vi "IMAQdx Enumerate Video Modes.vi"(8 "error in":errorcluster, 11 "Session In":T1) -> (0 "error out":errorcluster, 1 "Current Mode":u32, 2 "Video Modes":T2(array[cluster]), 3 "Session Out":T1)   [LabVIEW 2020, in "NI_Vision_Acquisition_Software.lvlib"]
doc: "Returns a list of video modes supported by the camera."
uses:
  NI_Vision_Acquisition_Software.lvlib
  IMAQdx.ctl
  niimaqdx.dll
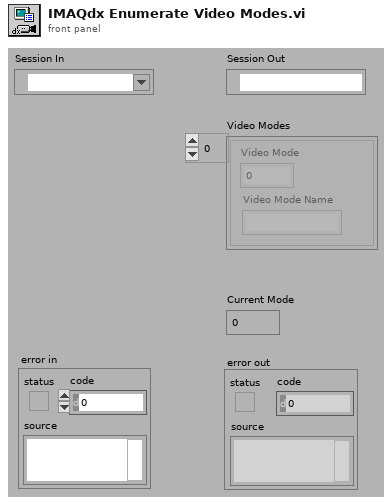
[diagram p1: front panel]
types:
  T1 = typedef "IMAQdx.ctl" = refnum<k21>
  T2 = cluster{"Video Mode":u32, "Video Mode Name":string}[]
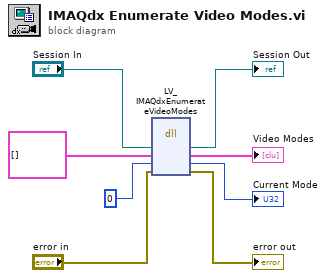
[diagram p0: block diagram]
diagram:
  n1 = dll-call lib="niimaqdx.dll" fn="LV_IMAQdxEnumerateVideoModes"("Session In"="Session In", "Video Modes"=T2 [], "currentMode"=u32 0, "error in"="error in") -> ("Session In"=→"Session Out":T1, "Video Modes"=→"Video Modes":T2, "currentMode"=→"Current Mode":u32, "error in"=→"error out":errorcluster)  [unwired: 4 in, 2 out]
